vi "initializeMission.vi"(4 "Tolerance (m)":dbl, 5 "Done":bool, 6 "Timeout (s)":dbl=-1.0, 7 "Duration (s)":dbl=-1.0, 8 "Error In":errorcluster, 9 "Points of Interest":T1[](array[typedef]) {"North" format="%#_10f"; "East" format="%#_8f"}, 10 "Mission Type":T2, 11 "Idle in":refnum<class "Idle.lvclass">) -> (0 "Error Out":errorcluster, 3 "Idle out":refnum<class "Idle.lvclass">)   [LabVIEW 2013, in "Idle.lvclass"]
doc: "This VI initializes a mission. Mission Type, Points of Interest, and Tolerance are required, and timeout and duration are both optional."
uses:
  trunk/Software/2-Think/2 Classes/Missions/Idle/Idle.lvclass
  Data/TypeDefs/MissionTypeControl.ctl
  GenericMission/GenericMission.lvclass
  Data/TypeDefs/UTM Location.ctl
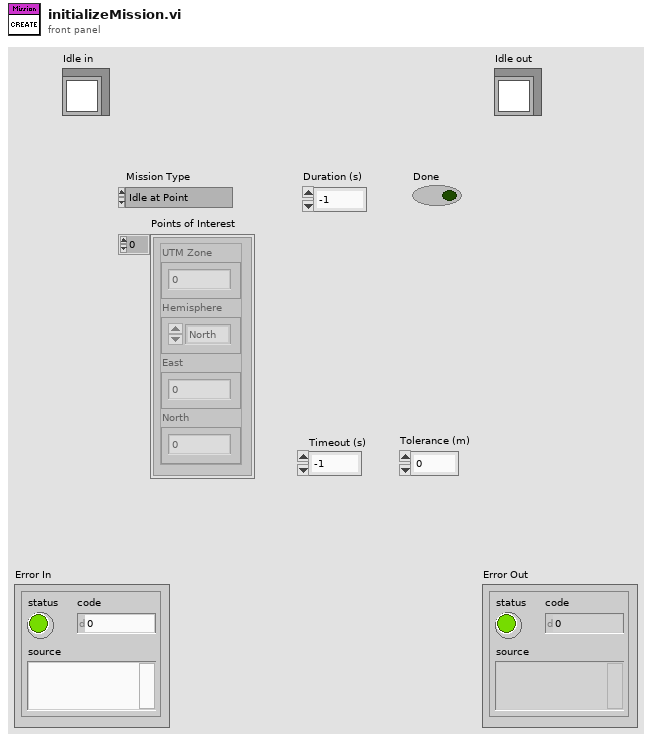
[diagram p1: front panel]
types:
  T1 = typedef "UTM Location.ctl" = cluster{"UTM Zone":dbl, "Hemisphere":enum16{"North", "South"}, "East":dbl, "North":dbl}
  T2 = typedef "MissionTypeControl.ctl" = enum16{"Idle at Point", "Drive to Waypoint", "Round Buoy to Port", "Round Buoy to Starboard", "Pass Between Buoys", "Station Keeping"}
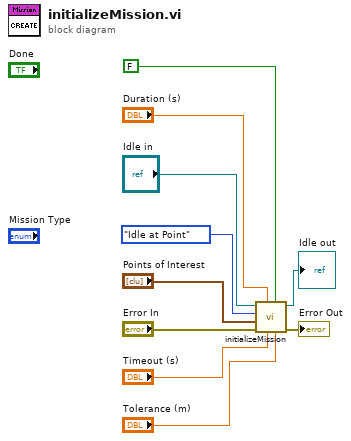
[diagram p0: block diagram]
diagram:
  n1 = call-parent "initializeMission.vi"("Tolerance (m)"="Tolerance (m)", "Done"=FALSE, "Timeout (s)"="Timeout (s)", "Duration (s)"="Duration (s)", "Error In"="Error In", "Points of Interest"="Points of Interest", "Mission Type"=MissionTypeControl."Idle at Point", "GenericMission in"="Idle in") -> ("Error Out"=→"Error Out":errorcluster, "GenericMission out"=→"Idle out":refnum<class "Idle.lvclass">)  [unwired: 2 in]
